vi "Ex6_Serrure_Num_2.vi"() -> ()   [LabVIEW 2018]
uses:
  Ex6_Serrure_Num_2_MDP.vi
panel:
  in  "stop":bool
  out "2D Picture":picture
  in  "BTN_Ouvrir":bool
  out "Max":u64
  out "Tentative":u64
  out "LED":bool
  in  "MDP_3":u16(knob)=1 max=9 scale=0.0..9.0
  in  "MDP_2":u16(knob)=1 max=9 scale=0.0..9.0
  in  "MDP_1":u16(knob)=1 max=9 scale=0.0..9.0
  # "/"
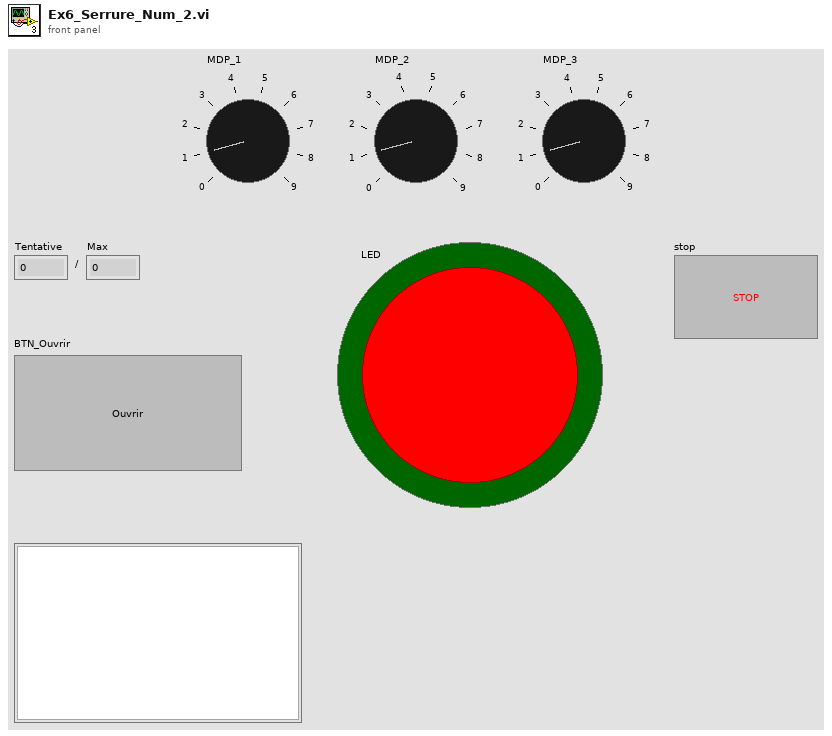
[diagram p1: front panel]
types:
  T1 = typedef "imagedata.ctl" = cluster{"image type":i32, "image depth":i32, "image":u8[], "mask":u8[], "colors":u32[], "Rectangle":cluster{"left":i16, "top":i16, "right":i16, "bottom":i16}}
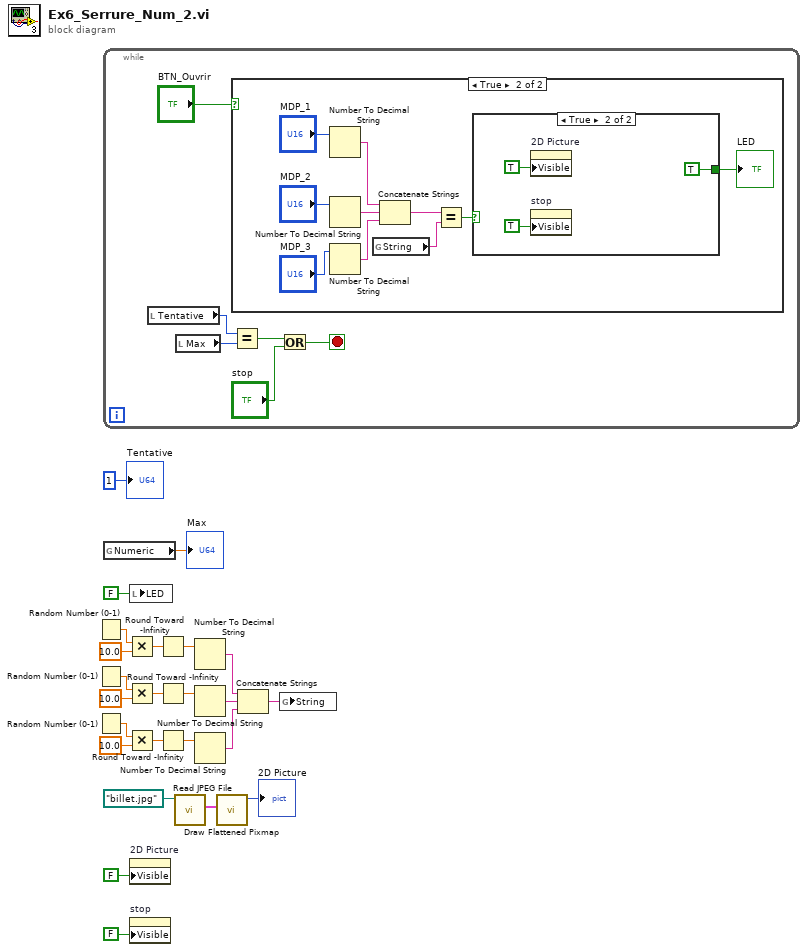
[diagram p0: block diagram]
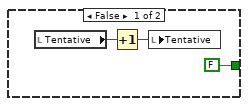
[diagram p3: hidden frame]
diagram:
  n1 = Random Number (0-1)() -> (number: 0 to 1=w19:dbl)
  n2 = Random Number (0-1)() -> (number: 0 to 1=w21:dbl)
  n3 = Random Number (0-1)() -> (number: 0 to 1=w18:dbl)
  n4 = while {
    stop <- w25 stop-if-true
    n5 = local read "Tentative"() -> (w30:u64)
    n6 = local read "Max"() -> (w29:u64)
    n7 = case shown="True" "BTN_Ouvrir" {
      frame False {
      }
      frame True {
        n8 = Number To Decimal String(number="MDP_1") -> (decimal integer string=w37:string)  [unwired: 1 in]
        n9 = Number To Decimal String(number="MDP_2") -> (decimal integer string=w36:string)  [unwired: 1 in]
        n10 = Number To Decimal String(number="MDP_3") -> (decimal integer string=w35:string)  [unwired: 1 in]
        n11 = global read "Ex6_Serrure_Num_2_MDP.vi" "String"() -> (w33:string)
        n12 = Concatenate Strings(w37, w36, w35) -> (w34:string)
        n13 = Equal?(x=w34, y=w33) -> (x = y?=w32:bool)
        n14 = case shown="True" w32 {
          tunnel: [FALSE TRUE] -> w31
          frame False {
            n15 = local read "Tentative"() -> (w42:u64)
            n16 = Increment(x=w42) -> (x+1=w41:u64)
            n17 = local write "Tentative"(w41) -> ()
          }
          frame True {
            n18 = property on="2D Picture" class="Pict"("Visible"=TRUE) -> ()  [unwired: 2 in, 2 out]
            n19 = property on="stop" class="Bool"("Visible"=TRUE) -> ()  [unwired: 2 in, 2 out]
          }
        }
        "LED" <- w31
      }
    }
    n20 = Equal?(x=w30, y=w29) -> (x = y?=w27:bool)
    n21 = Or(x=w27, y="stop") -> (x .or. y?=w25:bool)
  }
  n22 = global read "Ex6_Serrure_Num_2_MDP.vi" "Numeric"() -> (→"Max":dbl)
  n23 = Multiply(x=w19, y=10.0 ("x*y")) -> (x*y=w16:dbl)
  n24 = Multiply(x=w21, y=10.0) -> (x*y=w15:dbl)
  n25 = Multiply(x=w18, y=10.0 ("x*y")) -> (x*y=w14:dbl)
  n26 = local write "LED"(FALSE) -> ()
  n27 = property on="2D Picture" class="Pict"("Visible"=FALSE) -> ()  [unwired: 2 in, 2 out]
  n28 = property on="stop" class="Bool"("Visible"=FALSE) -> ()  [unwired: 2 in, 2 out]
  n29 = Round Toward -Infinity(1:w16) -> (0:w11:dbl)
  n30 = Round Toward -Infinity(1:w15) -> (0:w12:dbl)
  n31 = Round Toward -Infinity(1:w14) -> (0:w13:dbl)
  n32 = call <vilib>:"Read JPEG File.vi"("path to JPEG file"=path "billet.jpg") -> ("image data"=w5:T1)  [unwired: 8 in, 2 out]
  n33 = Number To Decimal String(number=w11) -> (decimal integer string=w10:string)  [unwired: 1 in]
  n34 = Number To Decimal String(number=w12) -> (decimal integer string=w9:string)  [unwired: 1 in]
  n35 = Number To Decimal String(number=w13) -> (decimal integer string=w8:string)  [unwired: 1 in]
  n36 = call <vilib>:"Draw Flattened Pixmap.vi"("image data"=w5) -> ("new picture"=→"2D Picture":picture)  [unwired: 8 in]
  n37 = Concatenate Strings(w10, w9, w8) -> (w7:string)
  n38 = global write "Ex6_Serrure_Num_2_MDP.vi" "String"(w7) -> ()
  "Tentative" <- u64 1 ("Tentative")
